vi "CreateG1Comm.vi"(1 "Numeric":dbl format="%#_13g", 2 "StartPoint":T1 {"U" format="%#.5g"; "X" format="%#.5g"; "Y" format="%#.5g"; "Z" format="%#.5g"}) -> (0 "String out":string)   [LabVIEW 2016]
uses:
  Control/Coordinate.ctl
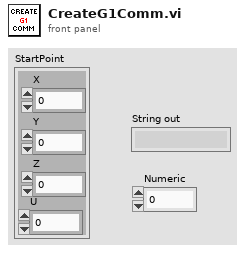
[diagram p1: front panel]
types:
  T1 = typedef "Coordinate.ctl" = cluster{"X":dbl, "Y":dbl, "Z":dbl, "U":dbl}
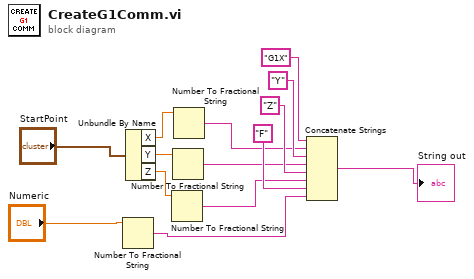
[diagram p0: block diagram]
diagram:
  n1 = Number To Fractional String(number="Numeric") -> (F-format string=w2:string)  [unwired: 3 in]
  n2 = Unbundle By Name("StartPoint") -> ("X"=w4:dbl, "Y"=w5:dbl, "Z"=w12:dbl)
  n3 = Number To Fractional String(number=w12) -> (F-format string=w11:string)  [unwired: 3 in]
  n4 = Number To Fractional String(number=w5) -> (F-format string=w7:string)  [unwired: 3 in]
  n5 = Number To Fractional String(number=w4) -> (F-format string=w6:string)  [unwired: 3 in]
  n6 = Concatenate Strings("G1X", w6, "Y", w7, "Z", w11, "F", w2) -> (→"String out":string)
